vi "Plot Scales GUI value change event.vi"(4 "NewVal":T2, 6 "OldVal":T2, 7 "Refs":T1, 8 "error in (no error)":errorcluster, 9 "Axis reference":refnum<vi>, 10 "Index":i32, 11 "axis SubRefs":T7) -> (0 "error out":errorcluster)   [LabVIEW 2021, in "RocketPlot.lvlib"]
uses:
  RocketPlot.lvlib
  TypeDefs/Plot axis GUI.ctl
  tick style/plot tick style picture ring.ctl
  lock/plot lock button.ctl
  horiz grid/plot horizontal grid pic ring.ctl
  vert grid/plot vertical grid pic ring.ctl
  TypeDefs/Plot axis gui refs.ctl
  TypeDefs/Plot UI references.ctl
  Classes/RocketPlotHandle/RocketPlotHandle.lvclass
  <userlib>/bjustice/TipStripOOPanel/Classes/TipPanelHandle/TipPanelHandle.lvclass
  TypeDefs/Plot top row.ctl
  Plot scale refnum to LUT name.vi
  FormatStringTime.vi
  Plot AxisFocus position.vi
  <vilib>/Utility/error.llb/Error Cluster From Error Code.vi
  <vilib>/ErrorRing/Error Ring.xnode
  <userlib>/_OpenG.lib/lvdata/lvdata.llb/openg_variant.lvlib
panel:
  # "Scaling Factors"
  # "Font Sizes"
  # "Scaling Factors"
  # "Font Sizes"
  # "Scaling Factors"
  # "Font Sizes"
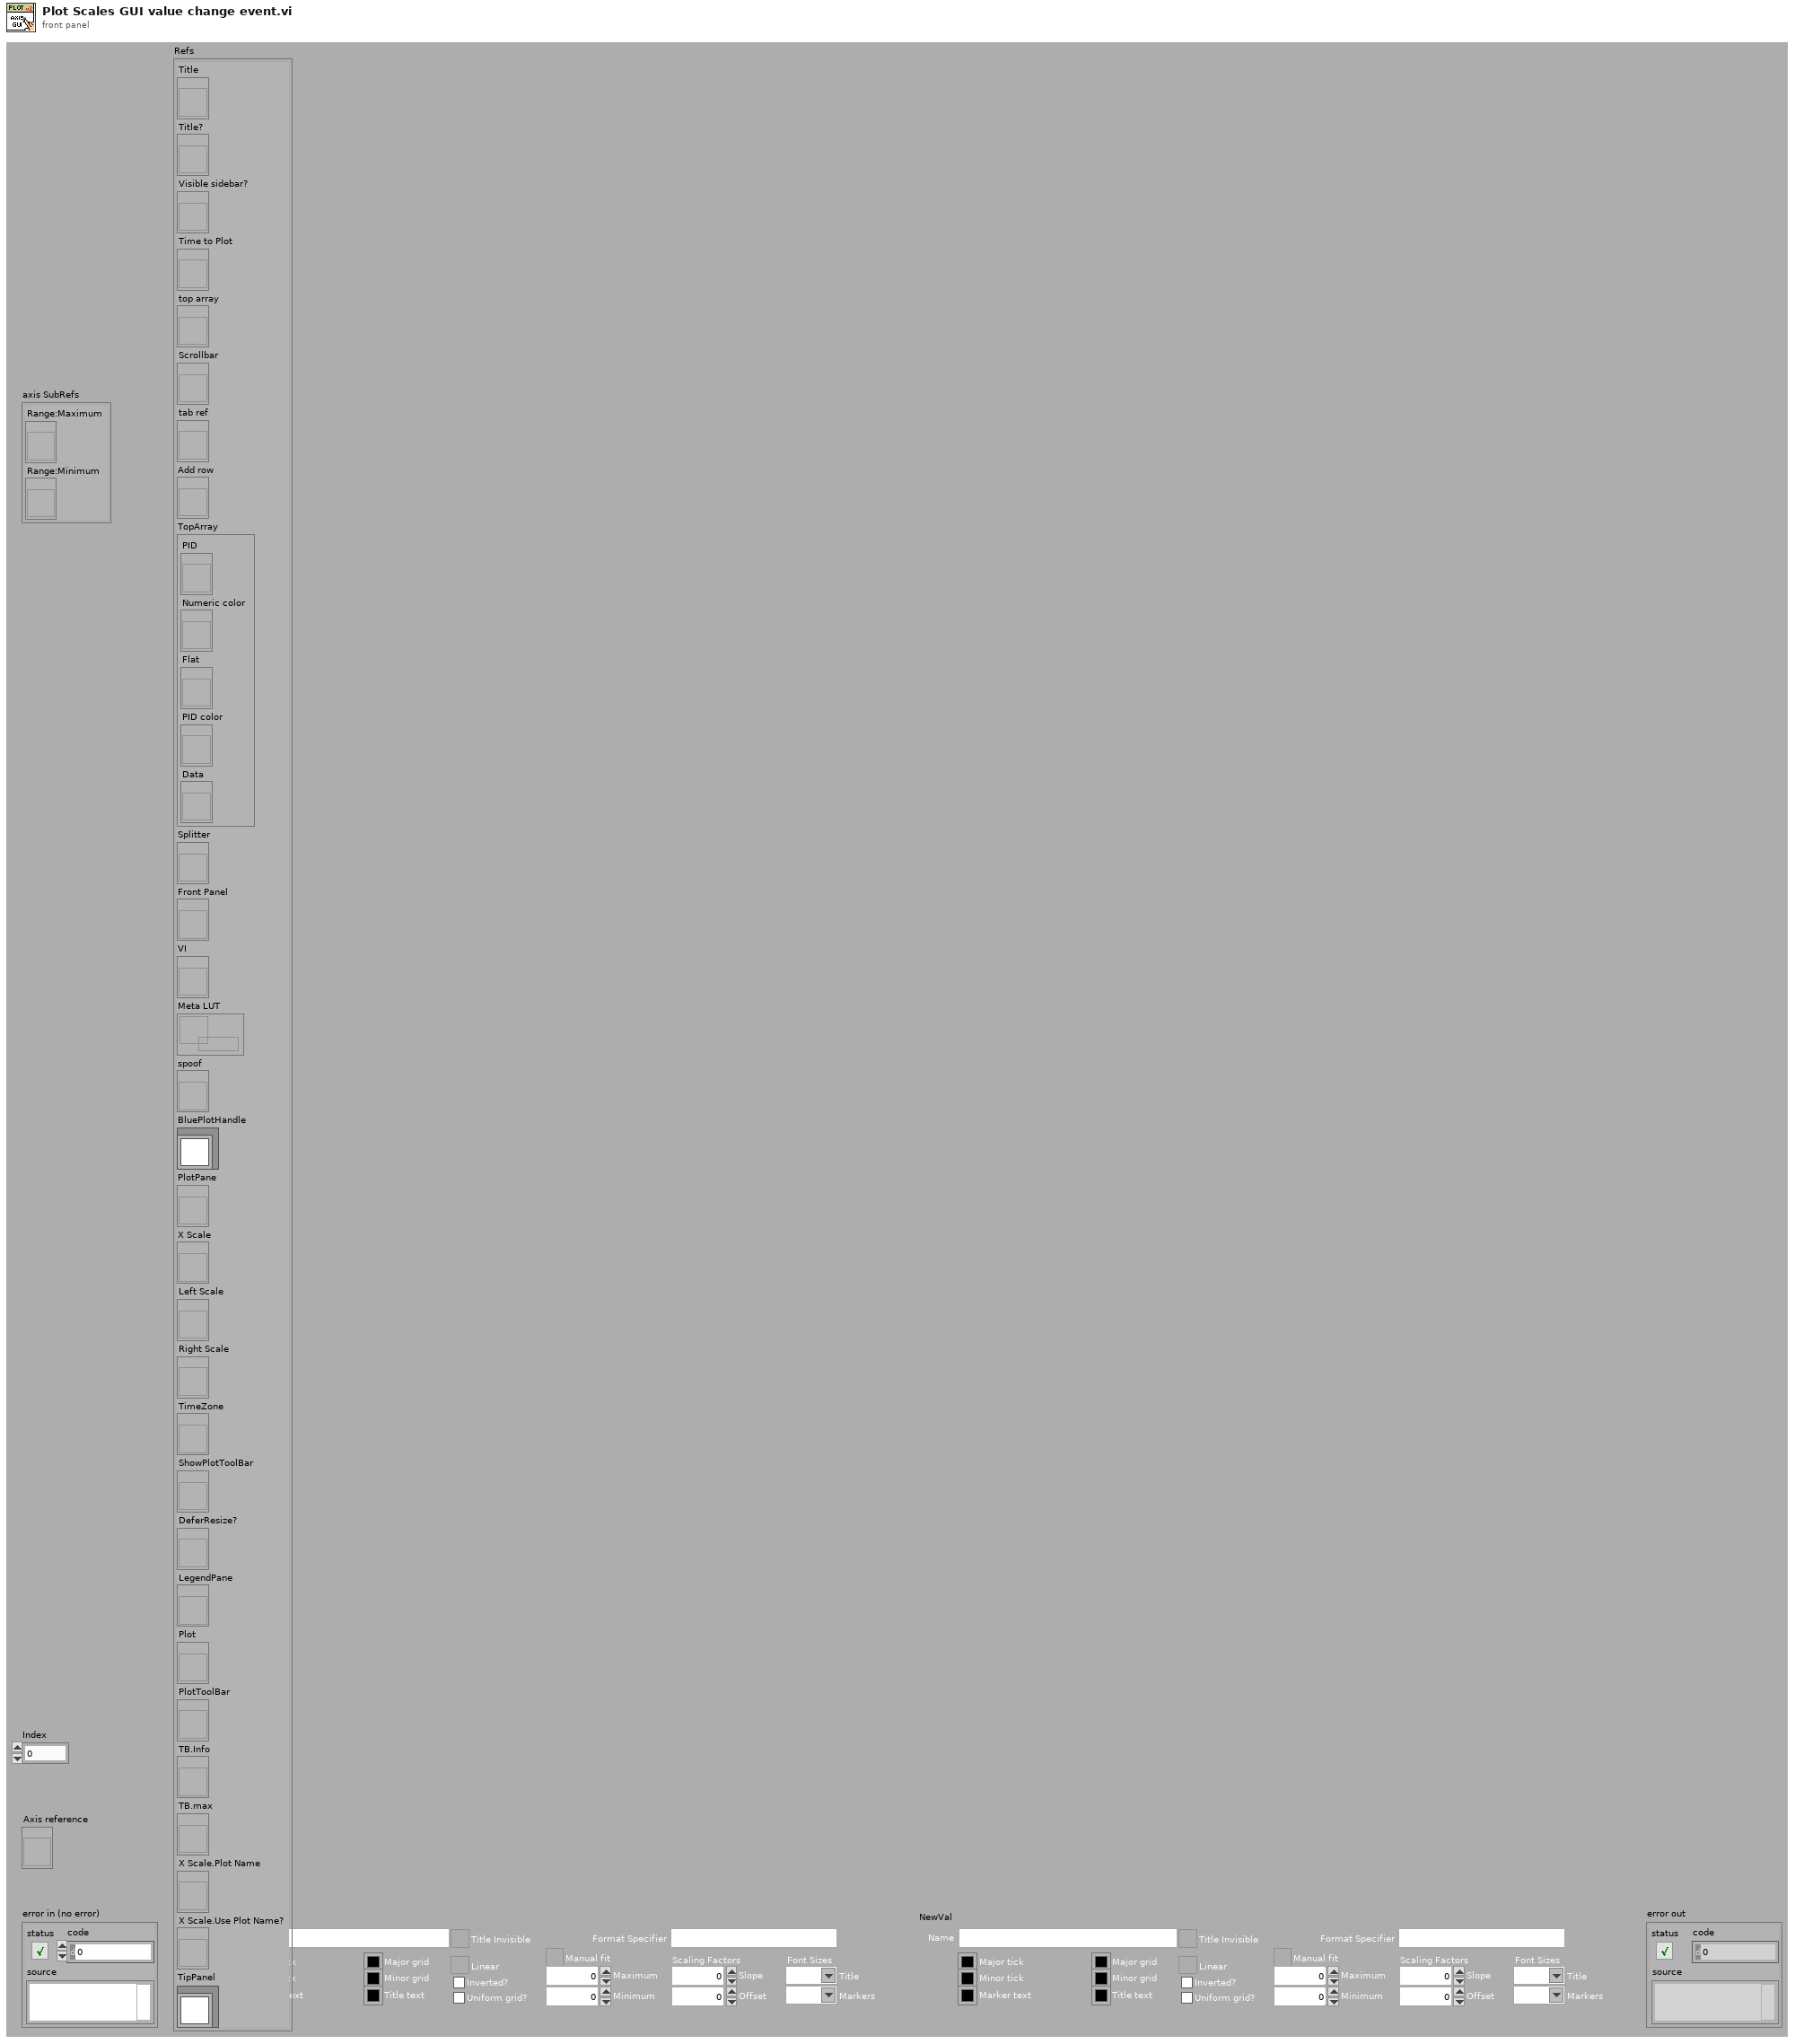
[diagram p1: front panel]
types:
  T1 = typedef "RocketPlot.lvlib/Plot UI references.ctl" = cluster{"Title":refnum<vi>, "Title?":refnum<vi>, "Visible sidebar?":refnum<vi>, "Time to Plot":refnum<vi>, "top array":refnum<vi>, "Scrollbar":refnum<vi>, "tab ref":refnum<vi>, "Add row":refnum<vi>, "TopArray":cluster{"PID":refnum<vi>, "Numeric color":refnum<vi>, "Flat":refnum<vi>, "PID color":refnum<vi>, "Data":refnum<vi>}, "Splitter":refnum<vi>, "Front Panel":refnum<vi>, "VI":refnum<vi>, "Meta LUT":refnum<data-value>, "spoof":refnum<vi>, "BluePlotHandle":refnum<class "RocketPlotHandle.lvclass">, "PlotPane":refnum<vi>, "X Scale":refnum<vi>, "Left Scale":refnum<vi>, "Right Scale":refnum<vi>, "TimeZone":refnum<vi>, "ShowPlotToolBar":refnum<vi>, "DeferResize?":refnum<vi>, "LegendPane":refnum<vi>, "Plot":refnum<vi>, "PlotToolBar":refnum<vi>, "TB.Info":refnum<vi>, "TB.max":refnum<vi>, "X Scale.Plot Name":refnum<vi>, "X Scale.Use Plot Name?":refnum<vi>, "TipPanel":refnum<class "TipPanelHandle.lvclass">}
  T2 = typedef "RocketPlot.lvlib/Plot axis GUI.ctl" = cluster{"Tick Colors:Tick Color":u32, "Tick Colors:Minor Tick Color":u32, "Name Label.Text":string, "Marker Colors:Text Color":u32, "Name Label.Font:Size":string, "Marker.Font:Size":string, "Flipped":bool, "Tick Style":T3, "Grid Colors:Major Color":u32, "Grid Colors:Minor Color":u32, "Mapping Mode":bool, "Autoscale?":T4, "Range:Minimum":dbl, "Range:Maximum":dbl, "Offset and Multiplier:Multiplier":dbl, "Offset and Multiplier:Offset":dbl, "Horiz.Grid Style":T5, "Name Label.Text Colors:Text Color":u32, "Vert.Grid Style":T6, "Name Label.Visible":bool, "Uniform Marker Spacing?":bool, "Format String":string}
  T3 = typedef "RocketPlot.lvlib/plot tick style picture ring.ctl" = u16
  T4 = typedef "RocketPlot.lvlib/plot lock button.ctl" = bool
  T5 = typedef "RocketPlot.lvlib/plot horizontal grid pic ring.ctl" = u16
  T6 = typedef "RocketPlot.lvlib/plot vertical grid pic ring.ctl" = u16
  T7 = typedef "RocketPlot.lvlib/Plot axis gui refs.ctl" = cluster{"Range:Maximum":refnum<vi>, "Range:Minimum":refnum<vi>}
  T8 = cluster{"Tick Colors:Tick Color":bool, "Tick Colors:Minor Tick Color":bool, "Name Label.Text":bool, "Marker Colors:Text Color":bool, "Name Label.Font:Size":bool, "Marker.Font:Size":bool, "Flipped":bool, "Tick Style":bool, "Grid Colors:Major Color":bool, "Grid Colors:Minor Color":bool, "Mapping Mode":bool, "Autoscale?":T4, "Range:Minimum":bool, "Range:Maximum":bool, "Offset and Multiplier:Multiplier":bool, "Offset and Multiplier:Offset":bool, "Horiz.Grid Style":bool, "Name Label.Text Colors:Text Color":bool, "Vert.Grid Style":bool, "Name Label.Visible":bool, "Uniform Marker Spacing?":bool, "Format String":bool}
  T9 = enum8{"Enabled", "Disabled", "Disabled and Grayed Out"}
  T10 = typedef "TimeZone.ctl" = enum16{"UTC", "Local"}
  T11 = typedef "RocketPlot.lvlib/Plot scale meta JSON.ctl" = cluster{"Type":T12, "Grid Colors:Major Color":u32, "Grid Colors:Minor Color":u32, "Style":u8, "Tick Colors:Tick Color":u32, "Tick Colors:Minor Tick Color":u32, "Format String":string, "State":T13, "AxisFocus":refnum<vi>}
  T12 = typedef "RocketPlot.lvlib/Plot axis.ctl" = enum16{"x axis", "left axis", "right axis"}
  T13 = typedef "RocketPlot.lvlib/Plot scale meta state.ctl" = cluster{"Visible":bool, "Focus":bool, "Multi-Y":bool}
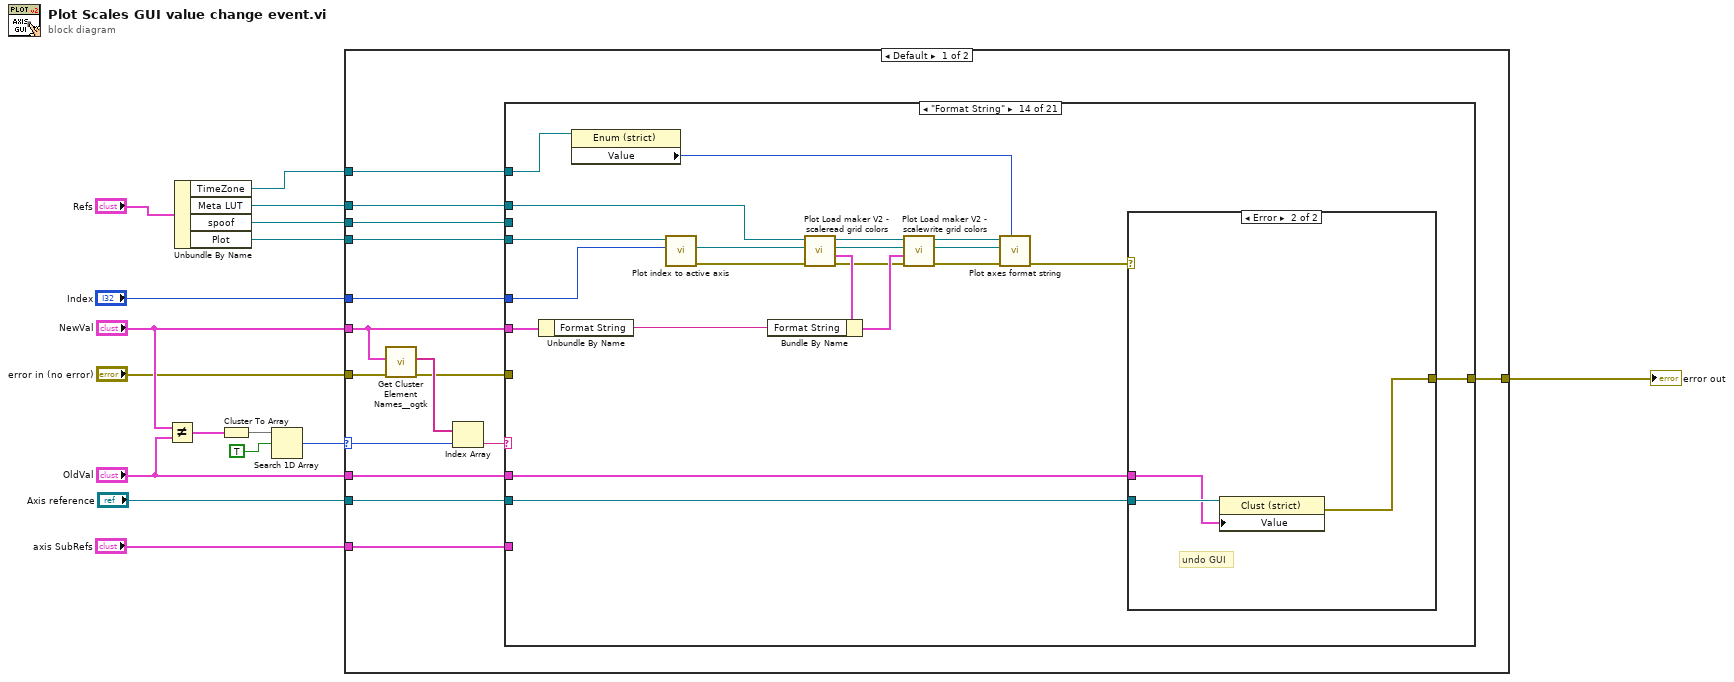
[diagram p0: block diagram]
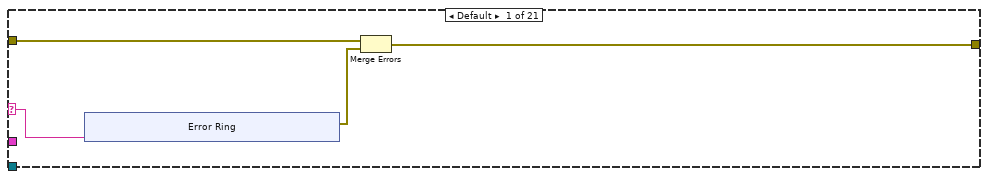
[diagram p2: hidden frame]
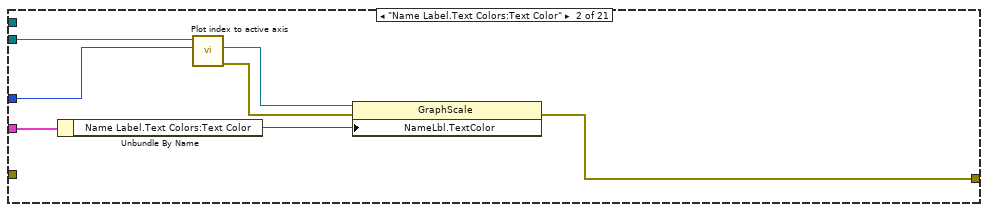
[diagram p3: hidden frame]
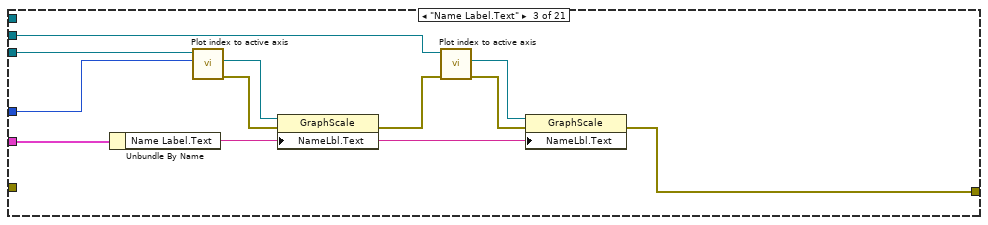
[diagram p4: hidden frame]
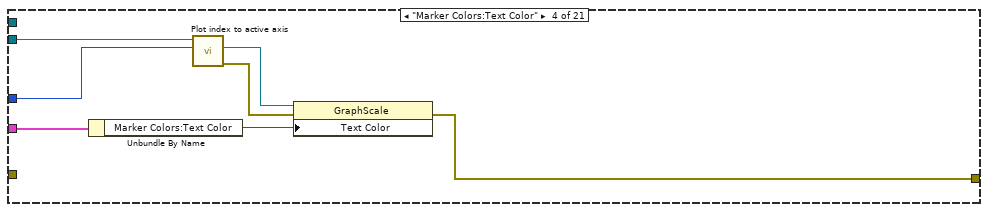
[diagram p5: hidden frame]
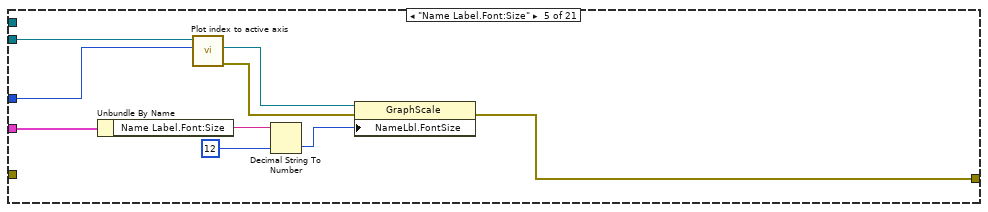
[diagram p6: hidden frame]
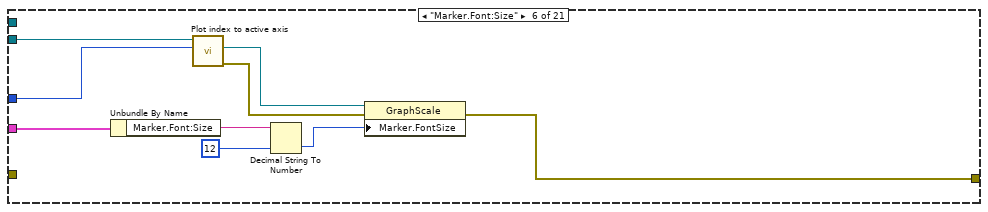
[diagram p7: hidden frame]
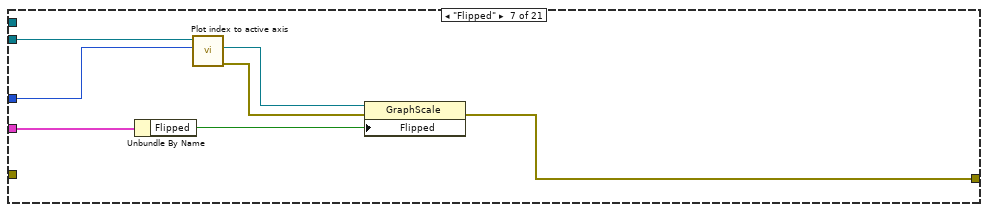
[diagram p8: hidden frame]
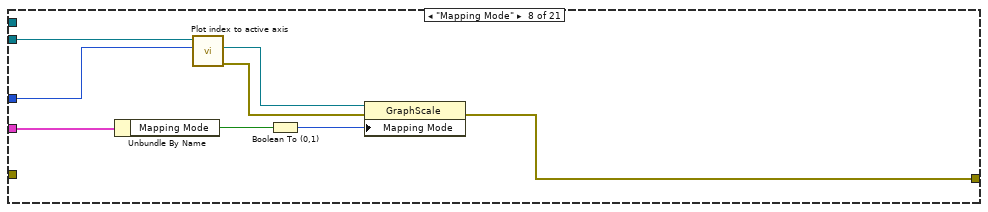
[diagram p9: hidden frame]
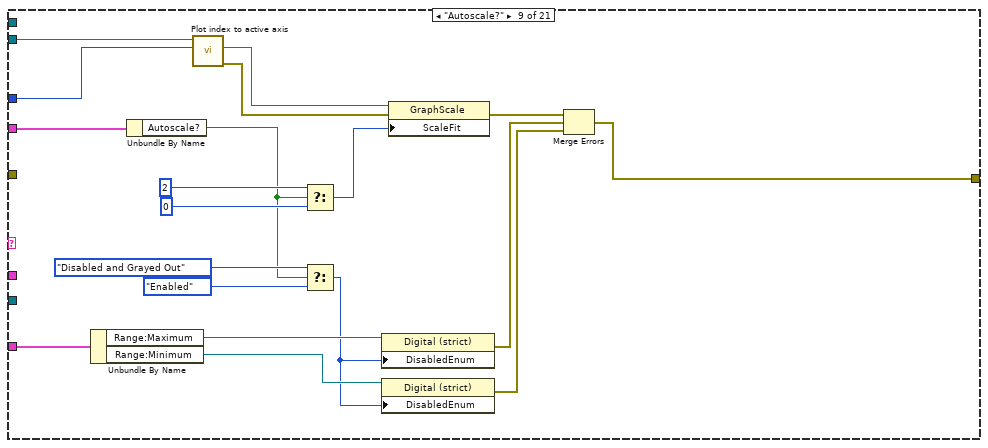
[diagram p10: hidden frame]
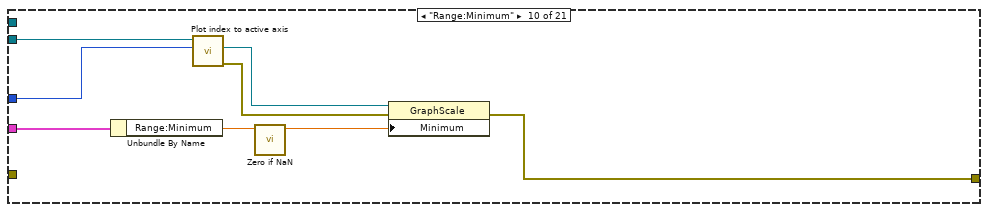
[diagram p11: hidden frame]
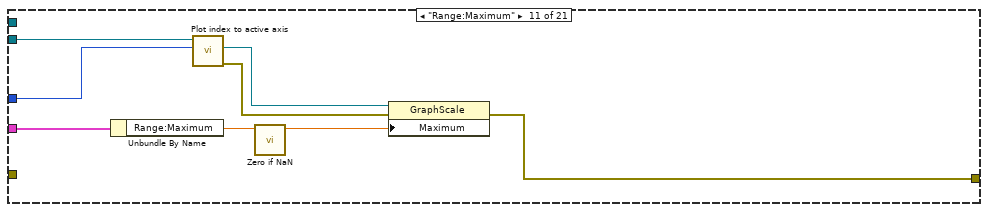
[diagram p12: hidden frame]
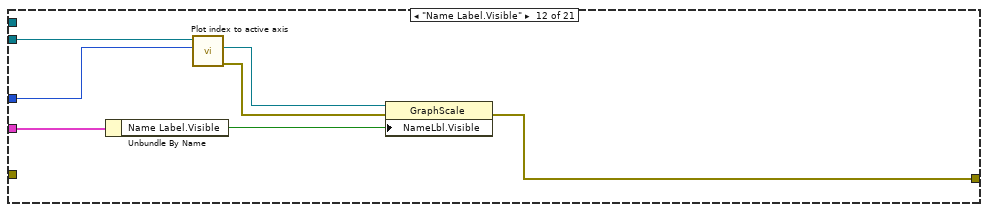
[diagram p13: hidden frame]
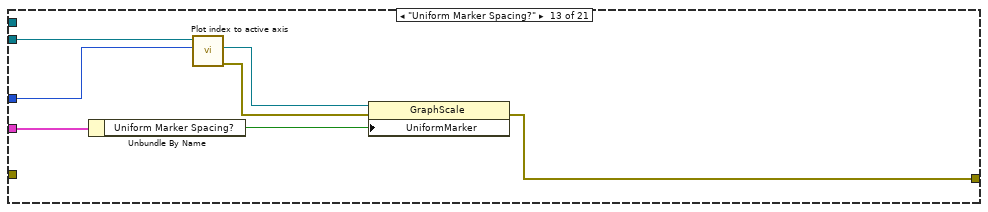
[diagram p14: hidden frame]
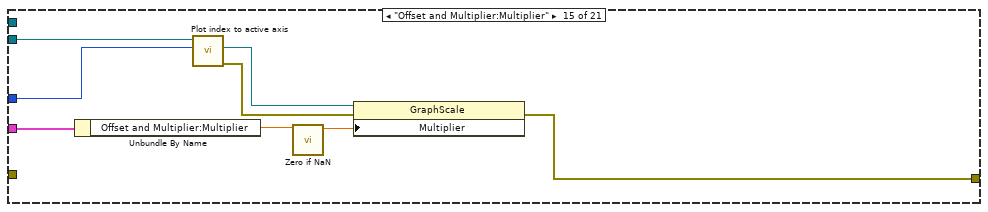
[diagram p16: hidden frame]
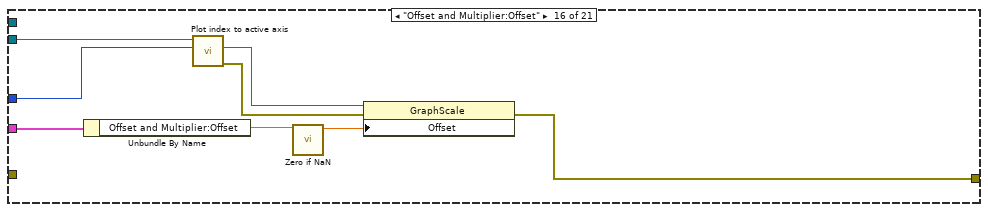
[diagram p17: hidden frame]
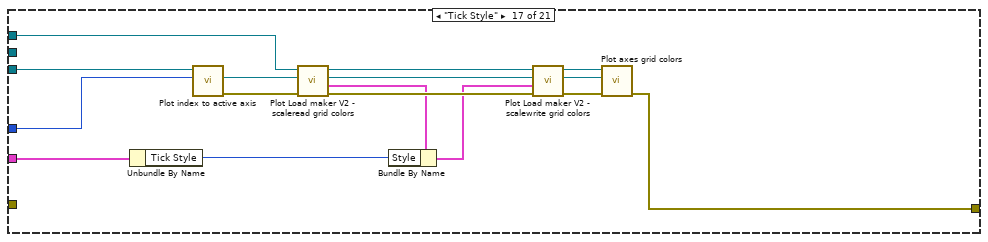
[diagram p18: hidden frame]
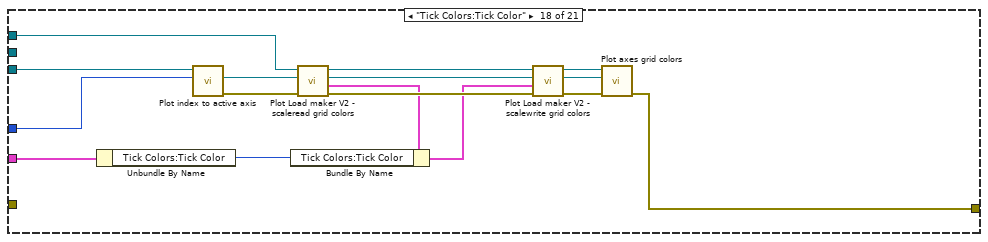
[diagram p19: hidden frame]
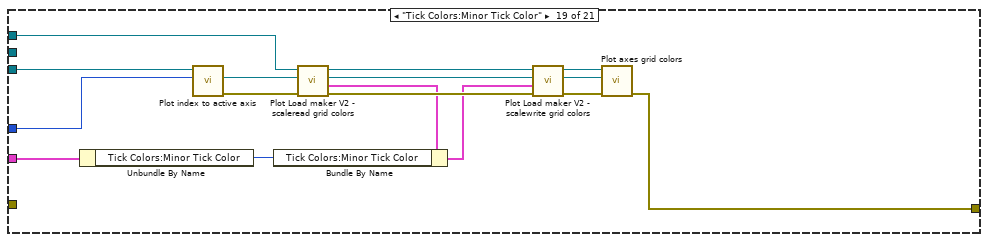
[diagram p20: hidden frame]
diagram:
  n1 = Not Equal?(x="NewVal", y="OldVal") -> (x != y?=w16:T8)
  n2 = Unbundle By Name("Refs") -> ("TimeZone"=w2:refnum<vi>, "Meta LUT"=w3:refnum<data-value>, "spoof"=w5:refnum<vi>, "Plot"=w9:refnum<vi>)
  n3 = Cluster To Array(cluster=w16) -> (array=w1:T4[])
  n4 = Search 1D Array(1D array=w1, element=TRUE) -> (index of element=w14:i32)  [unwired: 1 in]
  n5 = case shown="Default" w14 {
    selector: w14 -> [w30 _]
    tunnel: "NewVal" -> [w27 _]
    tunnel: "error in (no error)" -> [w26 w340]
    tunnel: [w25 w340] -> w11
    tunnel: w9 -> [w24 _]
    tunnel: "Index" -> [w23 _]
    tunnel: "axis SubRefs" -> [w22 _]
    tunnel: "Axis reference" -> [w21 _]
    tunnel: w5 -> [w20 _]
    tunnel: "OldVal" -> [w19 _]
    tunnel: w3 -> [w18 _]
    tunnel: w2 -> [w17 _]
    frame Default {
      n6 = call <userlib>:"Get Cluster Element Names__ogtk.vi"("error in (no error)"=w26, "Cluster"=w27) -> ("error out"=w28:errorcluster, "Element Names"=w31:string[])  [unwired: 8 in]
      n7 = Index Array(array=w31, index=w30) -> (element=w29:string)
      n8 = case shown="\"Format String\"" w29 {
        selector: w29 -> [w35 _ _ _ _ _ _ _ _ _ _ _ _ _ _ _ _ _ _ _ w261]
        tunnel: w28 -> [w34 _ _ _ _ _ _ _ _ _ _ _ _ _ _ _ _ _ _ _ _]
        tunnel: w27 -> [_ w49 w60 w67 w76 w85 w92 w100 w119 w127 w135 w142 w149 w170 w182 w190 w206 w222 w238 w255 w265]
        tunnel: [w32 w43 w50 w61 w71 w80 w87 w95 w103 w122 w130 w137 w144 w166 w177 w185 w191 w207 w223 w253 w267] -> w25
        tunnel: w24 -> [_ w48 w59 w66 w75 w84 w91 w99 w118 w126 w134 w141 w148 w169 w181 w189 w205 w221 w237 w259 w271]
        tunnel: w23 -> [_ w47 w58 w65 w74 w83 w90 w98 w117 w125 w133 w140 w147 w165 w180 w188 w204 w220 w236 w258 w270]
        tunnel: w22 -> [_ _ _ _ _ _ _ _ w112 _ _ _ _ _ _ _ _ _ _ _ _]
        tunnel: w21 -> [_ _ _ _ _ _ _ _ _ _ _ _ _ w168 _ _ _ _ _ w256 w264]
        tunnel: w20 -> [_ _ w55 _ _ _ _ _ _ _ _ _ _ _ _ _ _ _ _ _ _]
        tunnel: w19 -> [_ _ _ _ _ _ _ _ _ _ _ _ _ w167 _ _ _ _ _ _ _]
        tunnel: w18 -> [_ _ _ _ _ _ _ _ _ _ _ _ _ w157 _ _ w198 w214 w230 w244 w260]
        tunnel: w17 -> [_ _ _ _ _ _ _ _ _ _ _ _ _ w151 _ _ _ _ _ _ _]
        frame Default {
          n9 = xnode "Error Ring"("parameter 0"=w35) -> ("error out"=w33:errorcluster)
          n10 = Merge Errors(w34, w33) -> (w32:errorcluster)
        }
        frame "Name Label.Text Colors:Text Color" {
          n11 = Unbundle By Name(w49) -> ("Name Label.Text Colors:Text Color"=w45:u32)
          n12 = call "Plot index to active axis.vi"("Index"=w47, "Plot"=w48) -> ("error out"=w44:errorcluster, "Scale reference"=w46:refnum<vi>)  [unwired: 7 in, 1 out]
          n13 = property class="GraphScale"(reference=w46, error in=w44, "NameLbl.TextColor"=w45) -> (error out=w43:errorcluster)  [unwired: 1 out]
        }
        frame "Name Label.Text" {
          n14 = Unbundle By Name(w60) -> ("Name Label.Text"=w52:string)
          n15 = call "Plot index to active axis.vi"("Index"=w58, "Plot"=w59) -> ("error out"=w56:errorcluster, "Scale reference"=w57:refnum<vi>)  [unwired: 7 in, 1 out]
          n16 = property class="GraphScale"(reference=w57, error in=w56, "NameLbl.Text"=w52) -> (error out=w51:errorcluster)  [unwired: 1 out]
          n17 = call "Plot index to active axis.vi"("error in (no error)"=w51, "Plot"=w55) -> ("error out"=w54:errorcluster, "Scale reference"=w53:refnum<vi>)  [unwired: 7 in, 1 out]
          n18 = property class="GraphScale"(reference=w53, error in=w54, "NameLbl.Text"=w52) -> (error out=w50:errorcluster)  [unwired: 1 out]
        }
        frame "Marker Colors:Text Color" {
          n19 = Unbundle By Name(w67) -> ("Marker Colors:Text Color"=w63:u32)
          n20 = call "Plot index to active axis.vi"("Index"=w65, "Plot"=w66) -> ("error out"=w62:errorcluster, "Scale reference"=w64:refnum<vi>)  [unwired: 7 in, 1 out]
          n21 = property class="GraphScale"(reference=w64, error in=w62, "Text Color"=w63) -> (error out=w61:errorcluster)  [unwired: 1 out]
        }
        frame "Name Label.Font:Size" {
          n22 = Unbundle By Name(w76) -> ("Name Label.Font:Size"=w70:string)
          n23 = call "Plot index to active axis.vi"("Index"=w74, "Plot"=w75) -> ("error out"=w72:errorcluster, "Scale reference"=w73:refnum<vi>)  [unwired: 7 in, 1 out]
          n24 = Decimal String To Number(string=w70, default (0L)=u32 12 ("default (0 I32)")) -> (number=w68:u32)  [unwired: 1 in, 1 out]
          n25 = property class="GraphScale"(reference=w73, error in=w72, "NameLbl.FontSize"=w68) -> (error out=w71:errorcluster)  [unwired: 1 out]
        }
        frame "Marker.Font:Size" {
          n26 = Unbundle By Name(w85) -> ("Marker.Font:Size"=w79:string)
          n27 = call "Plot index to active axis.vi"("Index"=w83, "Plot"=w84) -> ("error out"=w81:errorcluster, "Scale reference"=w82:refnum<vi>)  [unwired: 7 in, 1 out]
          n28 = Decimal String To Number(string=w79, default (0L)=u32 12 ("default (0 I32)")) -> (number=w77:u32)  [unwired: 1 in, 1 out]
          n29 = property class="GraphScale"(reference=w82, error in=w81, "Marker.FontSize"=w77) -> (error out=w80:errorcluster)  [unwired: 1 out]
        }
        frame "Flipped" {
          n30 = Unbundle By Name(w92) -> ("Flipped"=w86:bool)
          n31 = call "Plot index to active axis.vi"("Index"=w90, "Plot"=w91) -> ("error out"=w88:errorcluster, "Scale reference"=w89:refnum<vi>)  [unwired: 7 in, 1 out]
          n32 = property class="GraphScale"(reference=w89, error in=w88, "Flipped"=w86) -> (error out=w87:errorcluster)  [unwired: 1 out]
        }
        frame "Mapping Mode" {
          n33 = Unbundle By Name(w100) -> ("Mapping Mode"=w94:bool)
          n34 = call "Plot index to active axis.vi"("Index"=w98, "Plot"=w99) -> ("error out"=w96:errorcluster, "Scale reference"=w97:refnum<vi>)  [unwired: 7 in, 1 out]
          n35 = Boolean To (0,1)(Boolean=w94) -> (0, 1=w93:i16)
          n36 = property class="GraphScale"(reference=w97, error in=w96, "Mapping Mode"=w93) -> (error out=w95:errorcluster)  [unwired: 1 out]
        }
        frame "Autoscale?" {
          n37 = Unbundle By Name(w112) -> ("Range:Maximum"=w111:refnum<vi>, "Range:Minimum"=w108:refnum<vi>)
          n38 = Unbundle By Name(w119) -> ("Autoscale?"=w101:T4)
          n39 = call "Plot index to active axis.vi"("Index"=w117, "Plot"=w118) -> ("error out"=w115:errorcluster, "Scale reference"=w116:refnum<vi>)  [unwired: 7 in, 1 out]
          n40 = Select(t=u8 2 ("Mapping Mode"), s=w101, f=u8 0 ("Mapping Mode")) -> (s? t:f=w102:u8)
          n41 = Select(t=T9."Disabled and Grayed Out" ("Disabled"), s=w101, f=T9."Enabled" ("Disabled")) -> (s? t:f=w107:T9)
          n42 = property class="Digital (strict)"(reference=w111, "DisabledEnum"=w107) -> (error out=w105:errorcluster)  [unwired: 1 in, 1 out]
          n43 = property class="Digital (strict)"(reference=w108, "DisabledEnum"=w107) -> (error out=w104:errorcluster)  [unwired: 1 in, 1 out]
          n44 = property class="GraphScale"(reference=w116, error in=w115, "ScaleFit"=w102) -> (error out=w106:errorcluster)  [unwired: 1 out]
          n45 = Merge Errors(w106, w105, w104) -> (w103:errorcluster)
        }
        frame "Range:Minimum" {
          n46 = Unbundle By Name(w127) -> ("Range:Minimum"=w121:dbl)
          n47 = call "Plot index to active axis.vi"("Index"=w125, "Plot"=w126) -> ("error out"=w123:errorcluster, "Scale reference"=w124:refnum<vi>)  [unwired: 7 in, 1 out]
          n48 = call "Zero if NaN.vi"("Numeric"=w121) -> ("Numeric"=w120:dbl)  [unwired: 10 in]
          n49 = property class="GraphScale"(reference=w124, error in=w123, "Minimum"=w120) -> (error out=w122:errorcluster)  [unwired: 1 out]
        }
        frame "Range:Maximum" {
          n50 = Unbundle By Name(w135) -> ("Range:Maximum"=w129:dbl)
          n51 = call "Plot index to active axis.vi"("Index"=w133, "Plot"=w134) -> ("error out"=w131:errorcluster, "Scale reference"=w132:refnum<vi>)  [unwired: 7 in, 1 out]
          n52 = call "Zero if NaN.vi"("Numeric"=w129) -> ("Numeric"=w128:dbl)  [unwired: 10 in]
          n53 = property class="GraphScale"(reference=w132, error in=w131, "Maximum"=w128) -> (error out=w130:errorcluster)  [unwired: 1 out]
        }
        frame "Name Label.Visible" {
          n54 = Unbundle By Name(w142) -> ("Name Label.Visible"=w136:bool)
          n55 = call "Plot index to active axis.vi"("Index"=w140, "Plot"=w141) -> ("error out"=w138:errorcluster, "Scale reference"=w139:refnum<vi>)  [unwired: 7 in, 1 out]
          n56 = property class="GraphScale"(reference=w139, error in=w138, "NameLbl.Visible"=w136) -> (error out=w137:errorcluster)  [unwired: 1 out]
        }
        frame "Uniform Marker Spacing?" {
          n57 = Unbundle By Name(w149) -> ("Uniform Marker Spacing?"=w143:bool)
          n58 = call "Plot index to active axis.vi"("Index"=w147, "Plot"=w148) -> ("error out"=w145:errorcluster, "Scale reference"=w146:refnum<vi>)  [unwired: 7 in, 1 out]
          n59 = property class="GraphScale"(reference=w146, error in=w145, "UniformMarker"=w143) -> (error out=w144:errorcluster)  [unwired: 1 out]
        }
        frame "Format String" {
          n60 = Unbundle By Name(w170) -> ("Format String"=w158:string)
          n61 = property class="Enum (strict)"(reference=w151) -> ("Value"=w150:T10)  [unwired: 1 in, 2 out]
          n62 = call "Plot index to active axis.vi"("Index"=w165, "Plot"=w169) -> ("error out"=w156:errorcluster, "Scale reference"=w159:refnum<vi>)  [unwired: 7 in, 1 out]
          n63 = call "Plot Load maker V2 - scaleread grid colors.vi"("error in (no error)"=w156, "Scale reference"=w159, "Meta LUT"=w157) -> ("error out"=w160:errorcluster, "Scale LUT meta"=w161:T11, "Scale reference"=w162:refnum<vi>, "Meta LUT"=w163:refnum<data-value>)  [unwired: 5 in]
          n64 = Bundle By Name(cluster=w161, "Format String"=w158) -> (w164:T11)
          n65 = call "Plot Load maker V2 - scalewrite grid colors.vi"("error in (no error)"=w160, "Meta"=w164, "Scale reference"=w162, "Meta LUT"=w163) -> ("error out"=w155:errorcluster, "Scale reference"=w153:refnum<vi>, "Meta LUT"=w154:refnum<data-value>)  [unwired: 5 in]
          n66 = call "Plot axes format string.vi"("TimeZone"=w150, "error in (no error)"=w155, "Scale reference"=w153, "Meta LUT"=w154) -> ("error out"=w152:errorcluster)  [unwired: 6 in, 1 out]
          n67 = case shown="Error" w152 {
            selector: w152 -> [w171 _]
            tunnel: w168 -> [_ w174]
            tunnel: w167 -> [_ w173]
            tunnel: [w171 w172] -> w166
            frame No Error {
            }
            frame Error {
              # "undo GUI"
              n68 = property class="Clust (strict)"(reference=w174, "Value"=w173) -> (error out=w172:errorcluster)  [unwired: 1 in, 1 out]
            }
          }
        }
        frame "Offset and Multiplier:Multiplier" {
          n69 = Unbundle By Name(w182) -> ("Offset and Multiplier:Multiplier"=w176:dbl)
          n70 = call "Plot index to active axis.vi"("Index"=w180, "Plot"=w181) -> ("error out"=w178:errorcluster, "Scale reference"=w179:refnum<vi>)  [unwired: 7 in, 1 out]
          n71 = call "Zero if NaN.vi"("Numeric"=w176) -> ("Numeric"=w175:dbl)  [unwired: 10 in]
          n72 = property class="GraphScale"(reference=w179, error in=w178, "Multiplier"=w175) -> (error out=w177:errorcluster)  [unwired: 1 out]
        }
        frame "Offset and Multiplier:Offset" {
          n73 = Unbundle By Name(w190) -> ("Offset and Multiplier:Offset"=w184:dbl)
          n74 = call "Plot index to active axis.vi"("Index"=w188, "Plot"=w189) -> ("error out"=w186:errorcluster, "Scale reference"=w187:refnum<vi>)  [unwired: 7 in, 1 out]
          n75 = call "Zero if NaN.vi"("Numeric"=w184) -> ("Numeric"=w183:dbl)  [unwired: 10 in]
          n76 = property class="GraphScale"(reference=w187, error in=w186, "Offset"=w183) -> (error out=w185:errorcluster)  [unwired: 1 out]
        }
        frame "Tick Style" {
          n77 = Unbundle By Name(w206) -> ("Tick Style"=w196:T3)
          n78 = call "Plot index to active axis.vi"("Index"=w204, "Plot"=w205) -> ("error out"=w200:errorcluster, "Scale reference"=w199:refnum<vi>)  [unwired: 7 in, 1 out]
          n79 = call "Plot Load maker V2 - scaleread grid colors.vi"("error in (no error)"=w200, "Scale reference"=w199, "Meta LUT"=w198) -> ("error out"=w203:errorcluster, "Scale LUT meta"=w197:T11, "Scale reference"=w201:refnum<vi>, "Meta LUT"=w202:refnum<data-value>)  [unwired: 5 in]
          n80 = Bundle By Name(cluster=w197, "Style"=w196) -> (w195:T11)
          n81 = call "Plot Load maker V2 - scalewrite grid colors.vi"("error in (no error)"=w203, "Meta"=w195, "Scale reference"=w201, "Meta LUT"=w202) -> ("error out"=w192:errorcluster, "Scale reference"=w193:refnum<vi>, "Meta LUT"=w194:refnum<data-value>)  [unwired: 5 in]
          n82 = call "Plot axes grid colors.vi"("error in (no error)"=w192, "Scale reference"=w193, "Meta LUT"=w194) -> ("error out"=w191:errorcluster)  [unwired: 6 in, 2 out]
        }
        frame "Tick Colors:Tick Color" {
          n83 = Unbundle By Name(w222) -> ("Tick Colors:Tick Color"=w212:u32)
          n84 = call "Plot index to active axis.vi"("Index"=w220, "Plot"=w221) -> ("error out"=w216:errorcluster, "Scale reference"=w215:refnum<vi>)  [unwired: 7 in, 1 out]
          n85 = call "Plot Load maker V2 - scaleread grid colors.vi"("error in (no error)"=w216, "Scale reference"=w215, "Meta LUT"=w214) -> ("error out"=w219:errorcluster, "Scale LUT meta"=w213:T11, "Scale reference"=w217:refnum<vi>, "Meta LUT"=w218:refnum<data-value>)  [unwired: 5 in]
          n86 = Bundle By Name(cluster=w213, "Tick Colors:Tick Color"=w212) -> (w211:T11)
          n87 = call "Plot Load maker V2 - scalewrite grid colors.vi"("error in (no error)"=w219, "Meta"=w211, "Scale reference"=w217, "Meta LUT"=w218) -> ("error out"=w208:errorcluster, "Scale reference"=w209:refnum<vi>, "Meta LUT"=w210:refnum<data-value>)  [unwired: 5 in]
          n88 = call "Plot axes grid colors.vi"("error in (no error)"=w208, "Scale reference"=w209, "Meta LUT"=w210) -> ("error out"=w207:errorcluster)  [unwired: 6 in, 2 out]
        }
        frame "Tick Colors:Minor Tick Color" {
          n89 = Unbundle By Name(w238) -> ("Tick Colors:Minor Tick Color"=w228:u32)
          n90 = call "Plot index to active axis.vi"("Index"=w236, "Plot"=w237) -> ("error out"=w232:errorcluster, "Scale reference"=w231:refnum<vi>)  [unwired: 7 in, 1 out]
          n91 = call "Plot Load maker V2 - scaleread grid colors.vi"("error in (no error)"=w232, "Scale reference"=w231, "Meta LUT"=w230) -> ("error out"=w235:errorcluster, "Scale LUT meta"=w229:T11, "Scale reference"=w233:refnum<vi>, "Meta LUT"=w234:refnum<data-value>)  [unwired: 5 in]
          n92 = Bundle By Name(cluster=w229, "Tick Colors:Minor Tick Color"=w228) -> (w227:T11)
          n93 = call "Plot Load maker V2 - scalewrite grid colors.vi"("error in (no error)"=w235, "Meta"=w227, "Scale reference"=w233, "Meta LUT"=w234) -> ("error out"=w224:errorcluster, "Scale reference"=w225:refnum<vi>, "Meta LUT"=w226:refnum<data-value>)  [unwired: 5 in]
          n94 = call "Plot axes grid colors.vi"("error in (no error)"=w224, "Scale reference"=w225, "Meta LUT"=w226) -> ("error out"=w223:errorcluster)  [unwired: 6 in, 2 out]
        }
        frame "Grid Colors:Major Color", "Grid Colors:Minor Color" {
          n95 = Unbundle By Name(w255) -> ("Grid Colors:Major Color"=w250:u32, "Grid Colors:Minor Color"=w252:u32)
          n96 = call "Plot index to active axis.vi"("Index"=w258, "Plot"=w259) -> ("error out"=w245:errorcluster, "Scale reference"=w243:refnum<vi>)  [unwired: 7 in, 1 out]
          n97 = call "Plot grid style TO.vi"("Grid Colors:Minor Color"=w252, "Grid Colors:Major Color"=w250) -> ("Grid Style"=w254:T5)  [unwired: 9 in]
          n98 = Bundle By Name(cluster=w255, "Horiz.Grid Style"=w254, "Vert.Grid Style"=w254) -> (w257:T2)
          n99 = call "Plot Load maker V2 - scaleread grid colors.vi"("error in (no error)"=w245, "Scale reference"=w243, "Meta LUT"=w244) -> ("error out"=w242:errorcluster, "Scale LUT meta"=w241:T11, "Scale reference"=w239:refnum<vi>, "Meta LUT"=w240:refnum<data-value>)  [unwired: 5 in]
          n100 = Bundle By Name(cluster=w241, "Grid Colors:Major Color"=w250, "Grid Colors:Minor Color"=w252) -> (w251:T11)
          n101 = call "Plot Load maker V2 - scalewrite grid colors.vi"("error in (no error)"=w242, "Meta"=w251, "Scale reference"=w239, "Meta LUT"=w240) -> ("error out"=w249:errorcluster, "Scale reference"=w248:refnum<vi>, "Meta LUT"=w247:refnum<data-value>)  [unwired: 5 in]
          n102 = call "Plot axes grid colors.vi"("error in (no error)"=w249, "Scale reference"=w248, "Meta LUT"=w247) -> ("error out"=w246:errorcluster)  [unwired: 6 in, 2 out]
          n103 = property class="Clust (strict)"(reference=w256, error in=w246, "Value"=w257) -> (error out=w253:errorcluster)  [unwired: 1 out]
        }
        frame "Horiz.Grid Style", "Vert.Grid Style" {
          n104 = case shown="\"Horiz.Grid Style\"" w261 {
            tunnel: [-1 w276 w280] -> w266
            tunnel: w265 -> [_ w275 w279]
            tunnel: [_ w274 w278] -> w263
            tunnel: [_ w273 w277] -> w262
            frame Default {
            }
            frame "Horiz.Grid Style" {
              n105 = Unbundle By Name(w275) -> ("Horiz.Grid Style"=w276:T5, "Grid Colors:Major Color"=w274:u32, "Grid Colors:Minor Color"=w273:u32)
            }
            frame "Vert.Grid Style" {
              n106 = Unbundle By Name(w279) -> ("Vert.Grid Style"=w280:T6, "Grid Colors:Major Color"=w278:u32, "Grid Colors:Minor Color"=w277:u32)
            }
          }
          n107 = call "Plot index to active axis.vi"("Index"=w270, "Plot"=w271) -> ("error out"=w268:errorcluster, "Scale reference"=w269:refnum<vi>)  [unwired: 7 in, 1 out]
          n108 = case shown="0..3" w266 {
            selector: w266 -> [w284 w306]
            tunnel: w269 -> [_ w294]
            tunnel: w268 -> [w283 w298]
            tunnel: [w281 w311] -> w267
            tunnel: w265 -> [_ w308]
            tunnel: w264 -> [_ w313]
            tunnel: w263 -> [_ w310]
            tunnel: w262 -> [_ w309]
            tunnel: w260 -> [_ w297]
            frame Default {
              n109 = xnode "Error Ring"("parameter 0"=w284) -> ("error out"=w282:errorcluster)
              n110 = Merge Errors(w283, w282) -> (w281:errorcluster)
            }
            frame 0..3 {
              n111 = case shown="0" w306 {
                tunnel: w310 -> [w315 w321 w327 w333 w339]
                tunnel: w309 -> [w314 w320 w326 w332 w338]
                tunnel: [w315 w319 w325 w331 w337] -> w305
                tunnel: [w314 w318 w324 w330 w336] -> w304
                frame Default {
                }
                frame 0 {
                  n112 = call "Plot default grid colors.vi"("Major Color visible?"=FALSE, "Minor Color visible?"=FALSE, "Minor Color"=w320, "Major Color"=w321) -> ("Minor Color"=w318:u32, "Major Color"=w319:u32)  [unwired: 6 in]
                }
                frame 1 {
                  n113 = call "Plot default grid colors.vi"("Major Color visible?"=TRUE, "Minor Color visible?"=FALSE, "Minor Color"=w326, "Major Color"=w327) -> ("Minor Color"=w324:u32, "Major Color"=w325:u32)  [unwired: 6 in]
                }
                frame 2 {
                  n114 = call "Plot default grid colors.vi"("Major Color visible?"=FALSE, "Minor Color visible?"=TRUE, "Minor Color"=w332, "Major Color"=w333) -> ("Minor Color"=w330:u32, "Major Color"=w331:u32)  [unwired: 6 in]
                }
                frame 3 {
                  n115 = call "Plot default grid colors.vi"("Major Color visible?"=TRUE, "Minor Color visible?"=TRUE, "Minor Color"=w338, "Major Color"=w339) -> ("Minor Color"=w336:u32, "Major Color"=w337:u32)  [unwired: 6 in]
                }
              }
              n116 = Bundle By Name(cluster=w308, "Grid Colors:Major Color"=w305, "Grid Colors:Minor Color"=w304) -> (w307:T2)
              n117 = call "Plot Load maker V2 - scaleread grid colors.vi"("error in (no error)"=w298, "Scale reference"=w294, "Meta LUT"=w297) -> ("error out"=w292:errorcluster, "Scale LUT meta"=w293:T11, "Scale reference"=w295:refnum<vi>, "Meta LUT"=w296:refnum<data-value>)  [unwired: 5 in]
              n118 = Bundle By Name(cluster=w293, "Grid Colors:Major Color"=w305, "Grid Colors:Minor Color"=w304) -> (w300:T11)
              n119 = call "Plot Load maker V2 - scalewrite grid colors.vi"("error in (no error)"=w292, "Meta"=w300, "Scale reference"=w295, "Meta LUT"=w296) -> ("error out"=w301:errorcluster, "Scale reference"=w302:refnum<vi>, "Meta LUT"=w303:refnum<data-value>)  [unwired: 5 in]
              n120 = property class="Clust (strict)"(reference=w313, "Value"=w307) -> (error out=w312:errorcluster)  [unwired: 1 in, 1 out]
              n121 = call "Plot axes grid colors.vi"("error in (no error)"=w301, "Scale reference"=w302, "Meta LUT"=w303) -> ("error out"=w299:errorcluster)  [unwired: 6 in, 2 out]
              n122 = Merge Errors(w299, w312) -> (w311:errorcluster)
            }
          }
        }
      }
    }
    frame -1 {
    }
  }
  "error out" <- w11
